vi "Get Sets Helper.vi"(6 "Item Types (all visible)":T4 items=["all visible", "all including hidden", "standard only", "startup only"], 8 "error in (no error)":errorcluster, 10 "Number of Elements":i32, 11 "Enumerator in":u64) -> (0 "error out":errorcluster, 2 "Software Sets":T1[](array[typedef]) {"information"."component type" items=["standard", "hidden", "system", "unknown", "startup", "image"]; "items"."component type" items=["standard", "hidden", "system", "unknown", "startup", "image"]; "add-ons"."component type" items=["standard", "hidden", "system", "unknown", "startup", "image"]}, 3 "Enumerator out":u64)   [LabVIEW 2014, in "nisyscfg.lvlib"]
uses:
  nisyscfg.lvlib
  Component Types.ctl
  Software Set 1.2.ctl
  Software 1.2.ctl
  Component Type.ctl
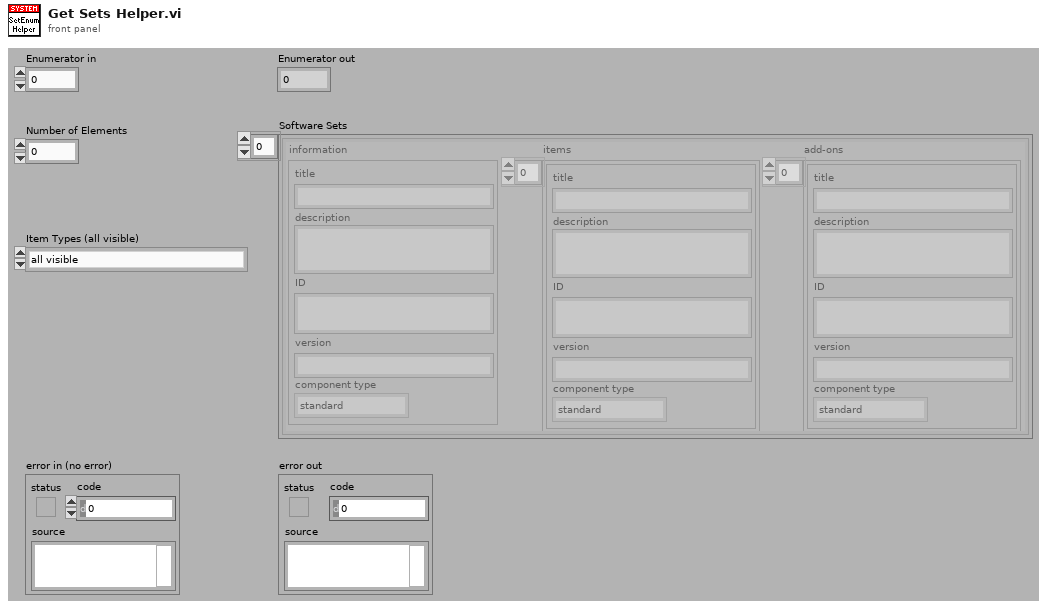
[diagram p1: front panel]
types:
  T1 = typedef "nisyscfg.lvlib/Software Set 1.2.ctl" = cluster{"information":T2, "items":T2[], "add-ons":T2[]}
  T2 = typedef "nisyscfg.lvlib/Software 1.2.ctl" = cluster{"title":string, "description":string, "ID":string, "version":string, "component type":T3}
  T3 = typedef "nisyscfg.lvlib/Component Type.ctl" = u32
  T4 = typedef "nisyscfg.lvlib/Component Types.ctl" = u32
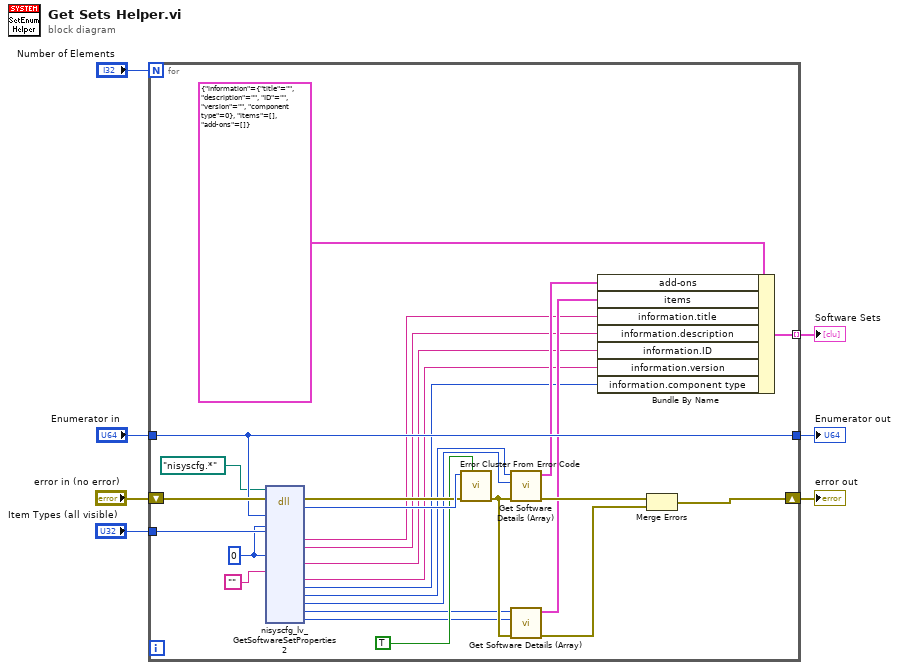
[diagram p0: block diagram]
diagram:
  n1 = for {
    N: "Number of Elements" -> [_]
    tunnel: "Enumerator in" -> [w21]
    shift-right: [w30] -> w4
    shift-left: "error in (no error)" -> [w33]
    tunnel: [w29] -> w1 mode=indexing
    tunnel: [w21] -> w6
    tunnel: "Item Types (all visible)" -> [w14]
    w13 = u8 0 ("includeAddOnDeps")
    n2 = dll-call lib="nisyscfg.*" fn="nisyscfg_lv_GetSoftwareSetProperties2" label="GetSoftwareSetProperties"(path in=path "nisyscfg.*", error in=w33, "setEnumerator"=w21, "includeAddOnDeps"=w13, "includeTypes"=w14, "type"=w13, "groupID"="") -> (error out=w31:errorcluster, "result"=w32:i32, "title"=w15:string, "description"=w16:string, "ID"=w12:string, "version"=w11:string, "visibleType"=w10:i32, "addons"=w26:u64, "numAddons"=w20:i32, "items"=w24:u64, "numItems"=w19:i32)  [unwired: 15 in, 1 out]
    n3 = call "Error Cluster From Error Code.vi"("show call chain? (False)"=TRUE, "error in (no error)"=w31, "error code (0)"=w32) -> ("error out"=w25:errorcluster)  [unwired: 6 in]
    n4 = call "Get Software Details (Array).vi"("error in (no error)"=w25, "Number of Elements"=w20, "Enumerator in"=w26) -> ("error out"=w23:errorcluster, "Software Components"=w18:T2[])  [unwired: 7 in]
    n5 = call "Get Software Details (Array).vi"("error in (no error)"=w25, "Number of Elements"=w19, "Enumerator in"=w24) -> ("error out"=w22:errorcluster, "Software Components"=w17:T2[])  [unwired: 7 in]
    n6 = Bundle By Name(cluster=T1 {"information"={"title"="", "description"="", "ID"="", "version"="", "component type"=0}, "items"=[], "add-ons"=[]} ("software set"), "add-ons"=w18, "items"=w17, "information.title"=w15, "information.description"=w16, "information.ID"=w12, "information.version"=w11, "information.component type"=w10) -> (w29:T1)
    n7 = Merge Errors(w23, w22) -> (w30:errorcluster)
  }
  "Enumerator out" <- w6
  "Software Sets" <- w1
  "error out" <- w4
